vi "DAQmx Write (Digital 2D Bool NChan 1Samp NLine).vi"(0 "task/channels in":refnum<k21>, 1 "auto start":bool=TRUE, 7 "data":bool[][](array[boolean]), 9 "timeout":dbl=10.0 format="%0.2f", 11 "error in":errorcluster) -> (4 "task out":refnum<k21>, 10 "number of samples written per channel":u32, 15 "error out":errorcluster)   [LabVIEW 2013]
doc: "Writes a single sample of Boolean values to each channel in a task that contains one or more digital output channels. The channels can contain one or more digital lines."
uses:
  nilvaiu.dll
panel:
  # "channel"
  # "line"
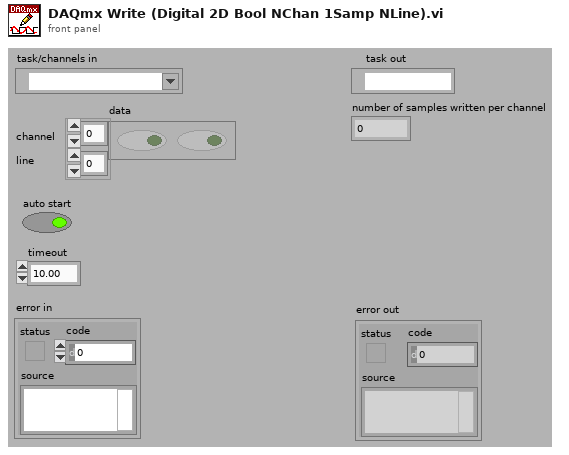
[diagram p1: front panel]
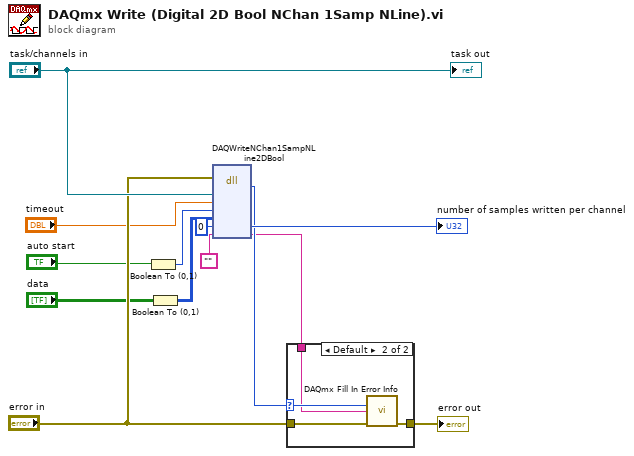
[diagram p0: block diagram]
diagram:
  n1 = Boolean To (0,1)(Boolean="auto start") -> (0, 1=w4:i16)
  n2 = Boolean To (0,1)(Boolean="data") -> (0, 1=w1:i16[][])
  n3 = dll-call lib="nilvaiu.*" fn="DAQWriteNChan1SampNLine2DBool"(error in="error in", "taskID"="task/channels in", "timeout"="timeout", "autoStart"=w4, "data"=w1, "numSamplesWriten"=u32 0, "extendedErrorInfo"="") -> (w6:i32, "numSamplesWriten"=→"number of samples written per channel":u32, "extendedErrorInfo"=w3:string)  [unwired: 3 in, 5 out]
  n4 = case shown="Default" w6 {
    selector: w6 -> [_ w16]
    tunnel: "error in" -> [w14 w18]
    tunnel: [w14 w17] -> w12
    tunnel: w3 -> [_ w15]
    frame 0 {
    }
    frame Default {
      n5 = call "DAQmx Fill In Error Info.vi"("status code"=w16, "extended error info"=w15, "error in"=w18) -> ("error out"=w17:errorcluster)  [unwired: 1 in, 11 out]
    }
  }
  "error out" <- w12
  "task out" <- "task/channels in"
